vi "Create Default User Config.vi"(8 "error in (no error)":errorcluster, 10 "User Config Path":path, 11 "App in":refnum<class "App.lvclass">) -> (0 "error out":errorcluster, 3 "App out":refnum<class "App.lvclass">)   [LabVIEW 2020, in "PicoG-App.lvlib" / "App.lvclass"]
uses:
  App.lvclass
  <vilib>/Utility/config.llb/NI_LVConfig.lvlib
  <vilib>/Utility/config.llb/Write Key (I32).vi
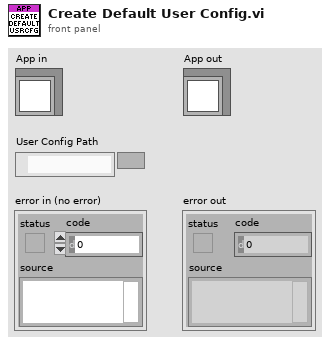
[diagram p1: front panel]
types:
  T1 = typedef "NI_LVConfig.lvlib/Config Data RefNum.ctl" = refnum<k1>
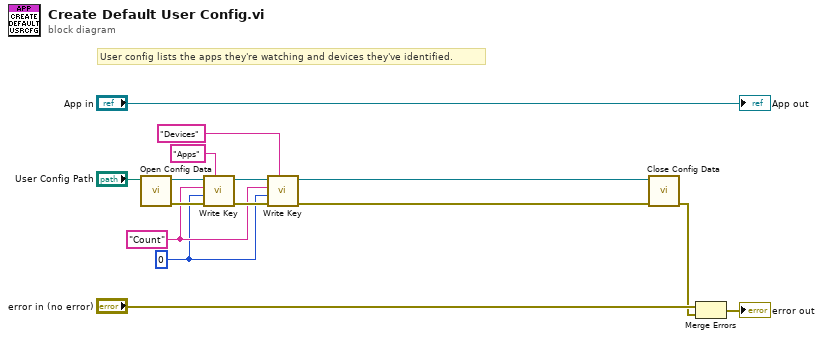
[diagram p0: block diagram]
diagram:
  w6 = 0 ("value")
  w7 = "Count"
  # "User config lists the apps they're watching and devices they've identified."
  n1 = call <vilib>:"Open Config Data.vi"("configuration file path"="User Config Path") -> ("error out"=w12:errorcluster, "refnum"=w13:T1)  [unwired: 8 in, 1 out]
  n2 = call-poly <vilib>:"Write Key.vi"("section"="Apps", "error in (no error)"=w12, "value"=w6, "key"=w7, "refnum"=w13) -> ("error out"=w10:errorcluster, "refnum out"=w11:T1)  [unwired: 4 in, 1 out]
  n3 = call-poly <vilib>:"Write Key.vi"("section"="Devices", "error in (no error)"=w10, "value"=w6, "key"=w7, "refnum"=w11) -> ("error out"=w4:errorcluster, "refnum out"=w5:T1)  [unwired: 4 in, 1 out]
  n4 = call <vilib>:"Close Config Data.vi"("error in (no error)"=w4, "refnum"=w5) -> ("error out"=w2:errorcluster)  [unwired: 8 in, 1 out]
  n5 = Merge Errors("error in (no error)", w2) -> (→"error out":errorcluster)
  "App out" <- "App in"
